vi "Shooter_Determiner.vi"() -> ()   [LabVIEW 2020]
uses:
  Shooter_Control_States.ctl
  Subsystems/Cowl/Cowl_Cluster.ctl
  Subsystems/Cowl/Cowl_States.ctl
  Subsystems/Turret/Turret_Cluster.ctl
  Subsystems/Turret/Turret_States.ctl
  Subsystems/Flywheel/Flywheel_Cluster.ctl
  Subsystems/Flywheel/Flywheel_States.ctl
  <vilib>/Rock Robotics/WPI/DriverStation/WPI_DriverStationRobotMode2.ctl
  Determiner_Begin_Cluster.ctl
  Shooter_Globals.vi
  Globals/Turret_Globals.vi
  Globals/Flywheel_Globals.vi
  Globals/Cowl_Globals.vi
  Robot Global Data.vi
panel:
  out "loop time":u32
  out "timed out?":bool
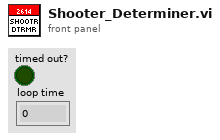
[diagram p1: front panel]
types:
  T1 = typedef "Shooter_Control_States.ctl" = enum16{"No-Op", "Limelight_Shooting", "Shoot_From_Pose", "Test"}
  T2 = typedef "WPI_DriverStationRobotMode2.ctl" = enum16{"Autonomous Disabled", "Autonomous Enabled", "Teleop Disabled", "Teleop Enabled", "Disconnected", "Finish", "Test Disabled", "Test Enabled", "Emergency Stopped"}
  T3 = typedef "Flywheel_Cluster.ctl" = cluster{"Flywheel_Throttle":dbl, "Flywheel_Control_State":T4, "Parameter_1":dbl, "Parameter_2":dbl, "Auto_Notifier":refnum<notifier>, "Step":dbl, "Flywheel_Velocity_Goal":dbl, "Flywheel_On ":bool}
  T4 = typedef "Flywheel_States.ctl" = enum16{"No-Op", "Percent_Voltage", "Speed_Control_Manual", "Speed_Control_Auto", "Command_SpinUp", "Command_SpinUpAuto"}
  T5 = typedef "Turret_Cluster.ctl" = cluster{"Turret_Control_State":T6, "Manual_Speed":dbl, "Step":dbl, "Parameter_1":dbl, "Parameter_2":dbl, "Parameter_3":dbl, "Auto_Notifier":refnum<notifier>, "Goal_Angle":dbl}
  T6 = typedef "Turret_States.ctl" = enum16{"Manual_Percent_Voltage", "Manual_Speed_Control", "Auto-Target", "Command_TurnToPosition", "Command_Auto_Target", "GoToZero", "No-Op"}
  T7 = typedef "Cowl_Cluster.ctl" = cluster{"Cowl_Control_State":T8, "Manual_Cowl_Throttle":dbl, "Cowl_Goal_Angle":dbl}
  T8 = typedef "Cowl_States.ctl" = enum16{"Manual_%VBus", "GoToAngle", "No-Op"}
  T9 = typedef "Determiner_Begin_Cluster.ctl" = cluster{"Shooter_Control_State":T1, "Shooting?":bool, "UpperGoal?":bool, "Limelight?":bool, "Flywheel_%Vbus":dbl, "Cowl_%Vbus":dbl, "Turret_%Vbus":dbl}
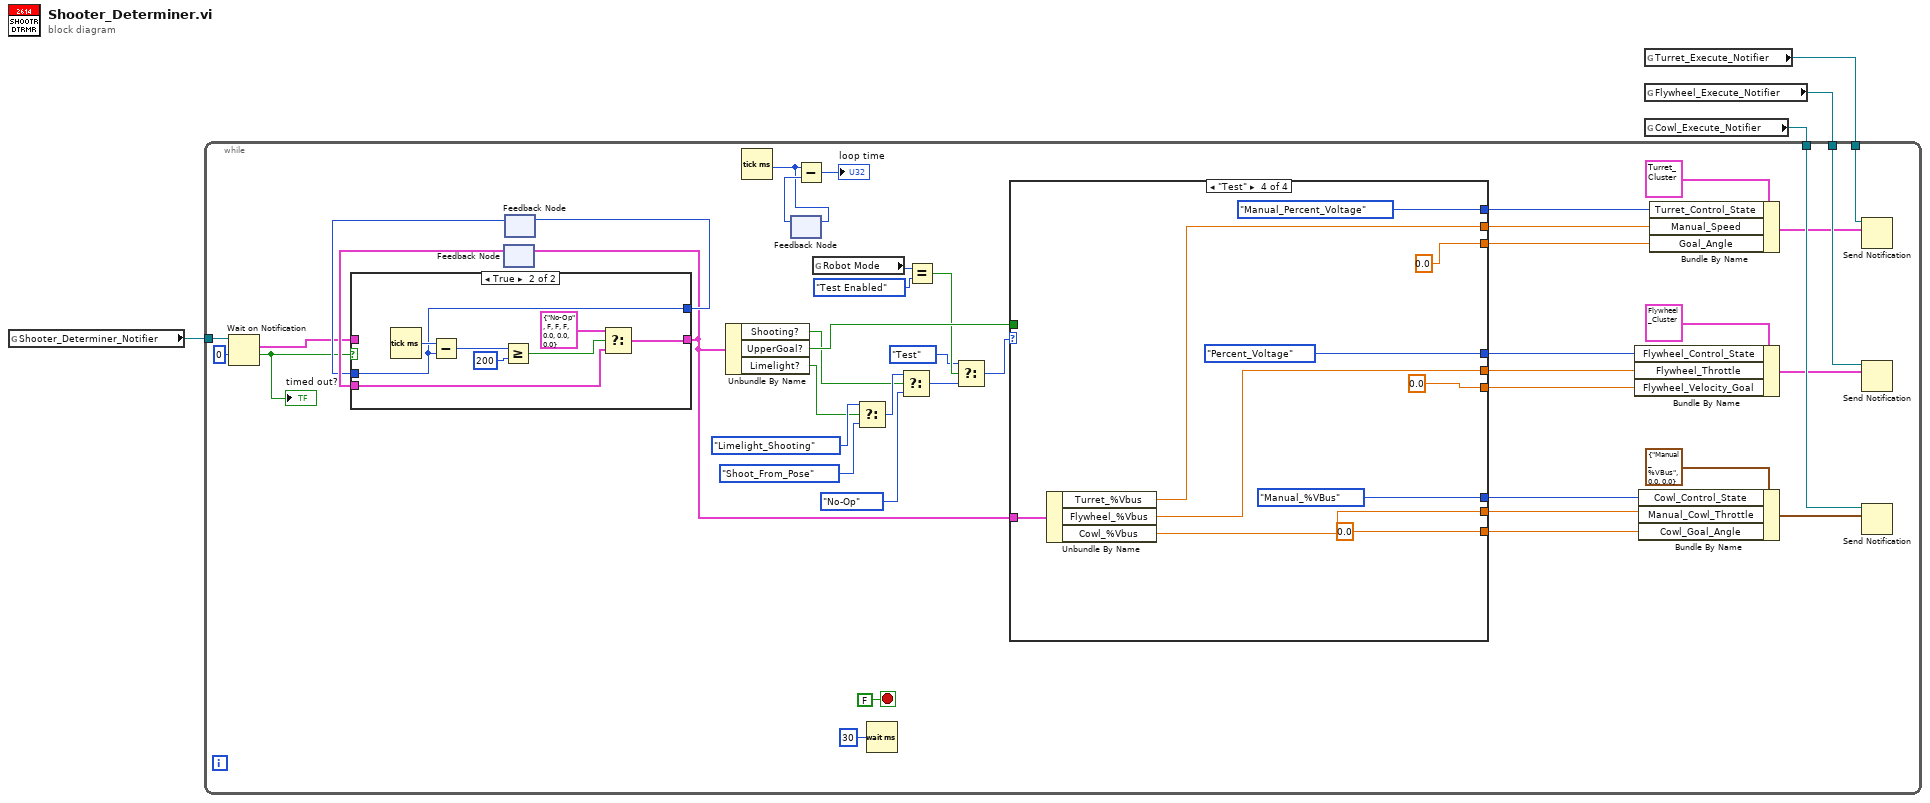
[diagram p0: block diagram]
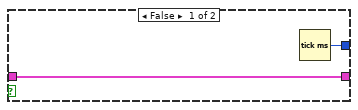
[diagram p2: hidden frame]
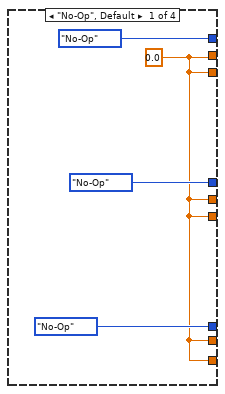
[diagram p3: hidden frame]
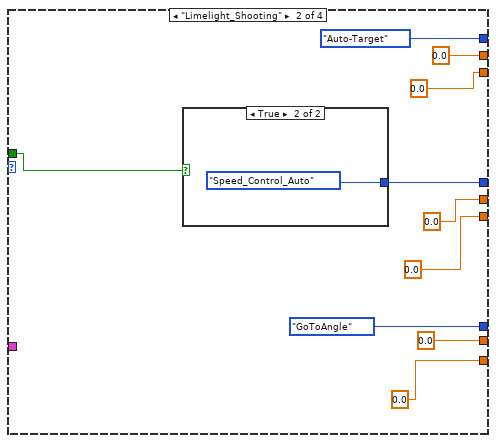
[diagram p4: hidden frame]
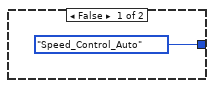
[diagram p5: hidden frame]
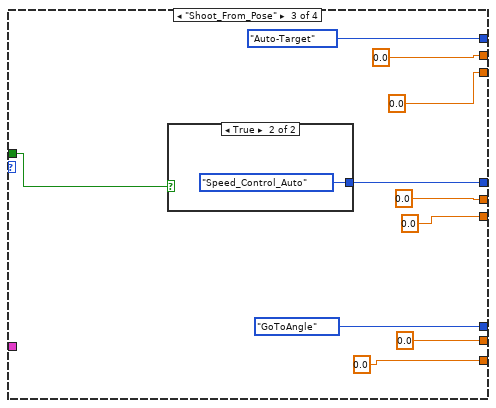
[diagram p6: hidden frame]
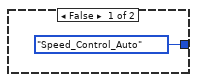
[diagram p7: hidden frame]
diagram:
  n1 = global read "Shooter_Globals.vi" "Shooter_Determiner_Notifier"() -> (w4:refnum<notifier>)
  n2 = global read "Turret_Globals.vi" "Turret_Execute_Notifier"() -> (w3:refnum<notifier>)
  n3 = global read "Flywheel_Globals.vi" "Flywheel_Execute_Notifier"() -> (w2:refnum<notifier>)
  n4 = global read "Cowl_Globals.vi" "Cowl_Execute_Notifier"() -> (w1:refnum<notifier>)
  n5 = while {
    tunnel: w4 -> [w48]
    tunnel: w3 -> [w28]
    tunnel: w2 -> [w30]
    tunnel: w1 -> [w29]
    stop <- FALSE stop-if-true
    n6 = Wait on Notification(notifier=w48, timeout in ms (-1)=0) -> (notification=w10:T9, timed out?=w9:bool)  [unwired: 2 in, 2 out]
    "timed out?" <- w9
    n7 = feedback #1() -> (w13:T9)  [unwired: 1 in]
    n8 = feedback #2() -> (w11:u32)  [unwired: 1 in]
    n9 = case shown="True" w9 {
      tunnel: w10 -> [w49 _]
      tunnel: [w49 w58] -> w6
      tunnel: w13 -> [_ w57]
      tunnel: [w50 w55] -> w12
      tunnel: w11 -> [_ w55]
      frame False {
        n10 = Tick Count (ms)() -> (millisecond timer value=w50:u32)
      }
      frame True {
        n11 = Tick Count (ms)() -> (millisecond timer value=w56:u32)
        n12 = Subtract(x=w56, y=w55) -> (x-y=w53:u32)
        n13 = Greater Or Equal?(x=w53, y=u32 200) -> (x >= y?=w54:bool)
        n14 = Select(t=T9 {"Shooter_Control_State"=enum."No-Op", "Shooting?"=FALSE, "UpperGoal?"=FALSE, "Limelight?"=FALSE, "Flywheel_%Vbus"=0.0, "Cowl_%Vbus"=0.0, "Turret_%Vbus"=0.0} ("notification"), s=w54, f=w57) -> (s? t:f=w58:T9)
      }
    }
    n15 = feedback-in #1(w6) -> ()
    n16 = feedback-in #2(w12) -> ()
    n17 = Unbundle By Name(w6) -> ("Shooting?"=w7:bool, "UpperGoal?"=w42:bool, "Limelight?"=w8:bool)
    n18 = Tick Count (ms)() -> (millisecond timer value=w16:u32)
    n19 = feedback-in #3(w16) -> ()
    n20 = feedback #3() -> (w17:u32)  [unwired: 1 in]
    n21 = Subtract(x=w16, y=w17) -> (x-y=→"loop time":u32)
    n22 = global read "Robot Global Data.vi" "Robot Mode"() -> (w23:T2)
    n23 = Select(t=Shooter_Control_States."Limelight_Shooting" ("Control_State"), s=w8, f=Shooter_Control_States."Shoot_From_Pose" ("Control_State")) -> (s? t:f=w43:T1)
    n24 = Wait (ms)(milliseconds to wait=u32 30) -> ()  [unwired: 1 out]
    n25 = Select(t=w43, s=w7, f=Shooter_Control_States."No-Op" ("Control_State")) -> (s? t:f=w21:T1)
    n26 = Equal?(x=w23, y=WPI_DriverStationRobotMode2."Test Enabled" ("Robot Mode")) -> (x = y?=w20:bool)
    n27 = Select(t=Shooter_Control_States."Test", s=w20, f=w21) -> (s? t:f=w22:T1)
    n28 = case shown="\"Test\"" w22 {
      tunnel: [Flywheel_States."No-Op" ("Control_States") w72 w84 Flywheel_States."Percent_Voltage" ("Control_States")] -> w33
      tunnel: [Turret_States."No-Op" ("Control_State") Turret_States."Auto-Target" ("Control_State") Turret_States."Auto-Target" ("Control_State") Turret_States."Manual_Percent_Voltage" ("Control_State")] -> w36
      tunnel: [Cowl_States."No-Op" ("Control_State") Cowl_States."GoToAngle" ("Cowl_Control_State") Cowl_States."GoToAngle" ("Cowl_Control_State") Cowl_States."Manual_%VBus" ("Cowl_Control_State")] -> w40
      tunnel: w42 -> [_ w63 w75 _]
      tunnel: [w59 0.0 0.0 0.0] -> w35
      tunnel: [w59 0.0 0.0 w88] -> w32
      tunnel: [w59 0.0 0.0 w89] -> w39
      tunnel: [w59 0.0 0.0 0.0] -> w38
      tunnel: [w59 0.0 0.0 w87] -> w14
      tunnel: [w59 0.0 0.0 0.0] -> w31
      tunnel: w6 -> [_ _ _ w90]
      frame "No-Op", Default {
        w59 = 0.0
      }
      frame "Limelight_Shooting" {
        n29 = case shown="True" w63 {
          tunnel: [Flywheel_States."Speed_Control_Auto" ("Flywheel_Control_State") Flywheel_States."Speed_Control_Auto" ("Flywheel_Control_State")] -> w72
          frame False {
          }
          frame True {
          }
        }
      }
      frame "Shoot_From_Pose" {
        n30 = case shown="True" w75 {
          tunnel: [Flywheel_States."Speed_Control_Auto" ("Flywheel_Control_State") Flywheel_States."Speed_Control_Auto" ("Flywheel_Control_State")] -> w84
          frame False {
          }
          frame True {
          }
        }
      }
      frame "Test" {
        n31 = Unbundle By Name(w90) -> ("Turret_%Vbus"=w87:dbl, "Flywheel_%Vbus"=w88:dbl, "Cowl_%Vbus"=w89:dbl)
      }
    }
    n32 = Bundle By Name(cluster=T3 {"Flywheel_Throttle"=0.0, "Flywheel_Control_State"=enum."No-Op", "Parameter_1"=0.0, "Parameter_2"=0.0, "Auto_Notifier"=refnum, "Step"=0.0, "Flywheel_Velocity_Goal"=0.0, "Flywheel_On "=FALSE} ("Flywheel_Cluster"), "Flywheel_Control_State"=w33, "Flywheel_Throttle"=w32, "Flywheel_Velocity_Goal"=w31) -> (w26:T3)
    n33 = Bundle By Name(cluster=T7 {"Cowl_Control_State"=enum."Manual_%VBus", "Manual_Cowl_Throttle"=0.0, "Cowl_Goal_Angle"=0.0} ("Cowl_Cluster"), "Cowl_Control_State"=w40, "Manual_Cowl_Throttle"=w39, "Cowl_Goal_Angle"=w38) -> (w25:T7)
    n34 = Bundle By Name(cluster=T5 {"Turret_Control_State"=enum."Manual_Percent_Voltage", "Manual_Speed"=0.0, "Step"=0.0, "Parameter_1"=0.0, "Parameter_2"=0.0, "Parameter_3"=0.0, "Auto_Notifier"=refnum, "Goal_Angle"=0.0} ("Turret_Cluster"), "Turret_Control_State"=w36, "Manual_Speed"=w14, "Goal_Angle"=w35) -> (w27:T5)
    n35 = Send Notification(notification=w27, notifier=w28) -> ()  [unwired: 1 in, 2 out]
    n36 = Send Notification(notification=w26, notifier=w30) -> ()  [unwired: 1 in, 2 out]
    n37 = Send Notification(notification=w25, notifier=w29) -> ()  [unwired: 1 in, 2 out]
  }
